vi "SURTENdll.vi"(8 "error in (no error)":errorcluster, 11 "Inputs":T2) -> (0 "error out":errorcluster, 3 "Outputs":T1)   [LabVIEW 2016]
doc: "subroutine SURTENdll(t, Dl, Dv, x, y, sigma, ierr, herr, herr_length)\n\nCompute surface tension\n\nINPUTS:\nt -- temperature [K]\nDl -- molar density of liquid phase [mol/L]\nDv -- molar density of vapor phase [mol/L]\n if either rhol or rhov < 0 call SATT to find densities\nx -- composition of liquid phase [array of mol frac]\ny -- composition of vapor phase [array of mol frac]\n (y is optional input if rhol < 0 or rhov < 0)\n\nOUTPUTS:\nsigma -- surface tension [N/m]\nierr -- error flag: 0 = successful\n 1 = T < Tmin\n 8 = x out of range\n 9 = T and x out of range\n 120 = CRITP did not converge\n 121 = T > Tcrit\n 122 = TPRHO-liquid did not converge in SATT\n 123 = TPRHO-vapor did not converge in SATT\n 124 = SATT pure fluid iteration did not converge\n 128 = SATT mixture iteration did not converge\nherr -- error string if ierr<>0 (character*255)\nherr_length -- length of variable herr (default: 255)"
uses:
  REFPROP.DLL
panel:
  # "REFPROP-SURTENdll.vi"
  # "void  SURTENdll(double *t, double *Dl, double *Dv, double *x, double *y, double *sigma, int32_t *ierr, CStr herr, int32_t herr_length)"
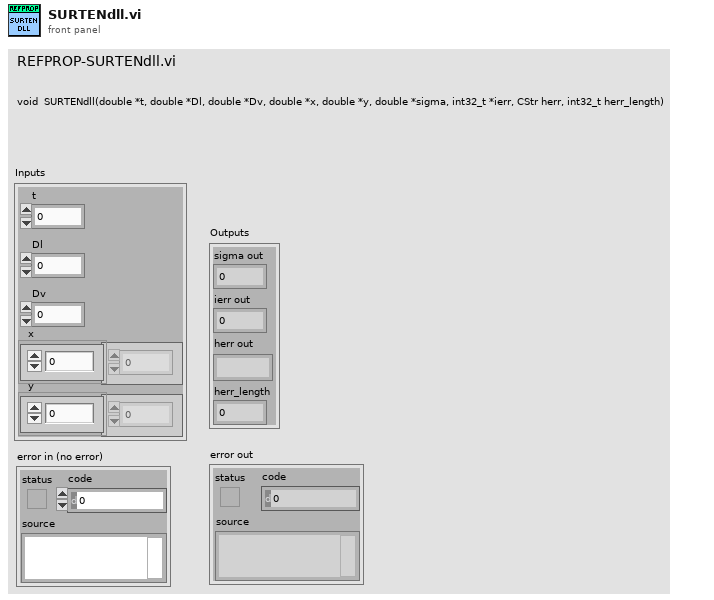
[diagram p1: front panel]
types:
  T1 = cluster{"sigma out":dbl, "ierr out":i32, "herr out":string, "herr_length":i32}
  T2 = cluster{"t":dbl, "Dl":dbl, "Dv":dbl, "x":dbl[], "y":dbl[]}
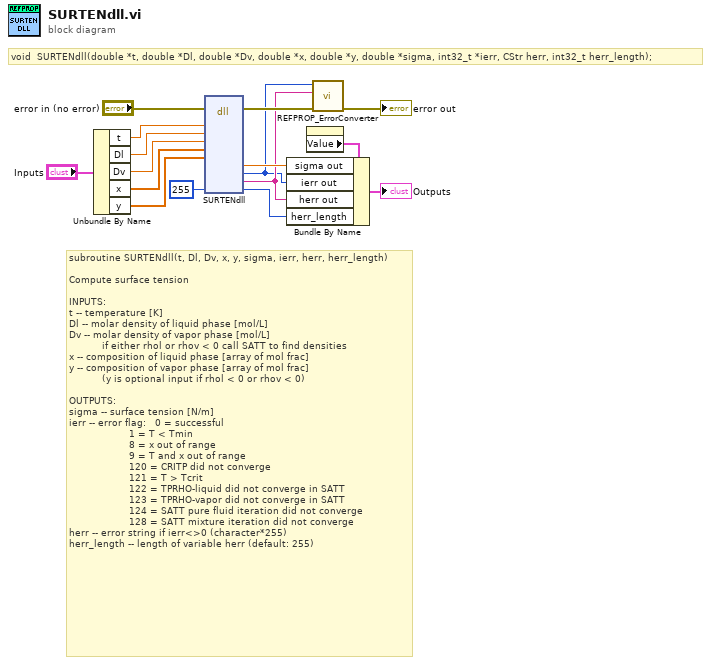
[diagram p0: block diagram]
diagram:
  # "void  SURTENdll(double *t, double *Dl, double *Dv, double *x, double *y, double *sigma, int32_t *ierr, CStr herr, int32_t herr_length);"
  # "subroutine SURTENdll(t, Dl, Dv, x, y, sigma, ierr, herr, herr_length)\n\nCompute surface tension\n\nINPUTS:\nt -- temperature [K]\nDl -- molar density of liquid phase [mol/L]\nDv -- molar density of vapor phase [mol/L]\n           if either rhol or rhov < 0 call SATT to find densities\nx -- composition of liquid phase [array of mol frac]\ny -- composition of vapor phase [array of mol frac]\n           (y is optional input if rhol < 0 or rhov < 0)\n\nOUTPUTS:\nsigma -- surface tension [N/m]\nierr -- error flag:   0 = successful\n                    1 = T < Tmin\n                    8 = x out of range\n                    9 = T and x out of range\n                    120 = CRITP did not converge\n                    121 = T > Tcrit\n                    122 = TPRHO-liquid did not converge in SATT\n                    123 = TPRHO-vapor did not converge in SATT\n                    124 = SATT pure fluid iteration did not converge\n                    128 = SATT mixture iteration did not converge\nherr -- error string if ierr<>0 (character*255)\nherr_length -- length of variable herr (default: 255)"
  n1 = Unbundle By Name("Inputs") -> ("t"=w11:dbl, "Dl"=w10:dbl, "Dv"=w9:dbl, "x"=w8:dbl[], "y"=w7:dbl[])
  n2 = dll-call lib="S:/009 - Testing/02 - Performance Testing/REFPROP/REFPROP.*" fn="SURTENdll"(error in="error in (no error)", "t"=w11, "Dl"=w10, "Dv"=w9, "x"=w8, "y"=w7, "herr_length"=255) -> (error out=w15:errorcluster, "sigma"=w5:dbl, "ierr"=w1:i32, "herr"=w2:string, "herr_length"=w4:i32)  [unwired: 11 in, 1 out]
  n3 = property on="Outputs" class="Clust (strict)"() -> ("Value"=w6:T1)  [unwired: 2 in, 2 out]
  n4 = Bundle By Name(cluster=w6, "sigma out"=w5, "ierr out"=w1, "herr out"=w2, "herr_length"=w4) -> (→"Outputs":T1)
  n5 = call "REFPROP_ErrorConverter.vi"("error in (no error)"=w15, "Error Message"=w2, "Error Code"=w1) -> ("error out"=→"error out":errorcluster)  [unwired: 8 in]
